vi "Simulated-acquisition-loop.vi"(4 "Timeout":timestamp, 6 "Acquisition notif":refnum<notifier>, 8 "error in (no error)":errorcluster, 9 "Buffers":refnum<class "CV-Buffers.lvclass">, 10 "Config. params. ref. in":refnum<data-value>, 11 "Acquis. params. ref. in":refnum<data-value>) -> (0 "error out":errorcluster, 2 "Config. params. ref.":refnum<data-value>, 3 "Acquis. params. ref.":refnum<data-value>)   [LabVIEW 2013, in "CameraVision.lvlib" / "CV-Acquisition.lvclass"]
uses:
  CV-Acquisition.lvclass
  Configuration/CV-Configuration.lvclass
  Buffers/CV-Buffers.lvclass
  <vilib>/Platform/TimedLoop/XDataNode/timing_clust.ctl
  <vilib>/Platform/TimedLoop/XDataNode/nitl_modes.ctl
  <vilib>/Platform/TimedLoop/XDataNode/wakeup.ctl
  <vilib>/Platform/TimedLoop/XDataNode/XDataNode.xnode
  <vilib>/Platform/TimedLoop/XDataNode/XDNodeRunTimeDep.lvlib
  CV-Main.lvclass
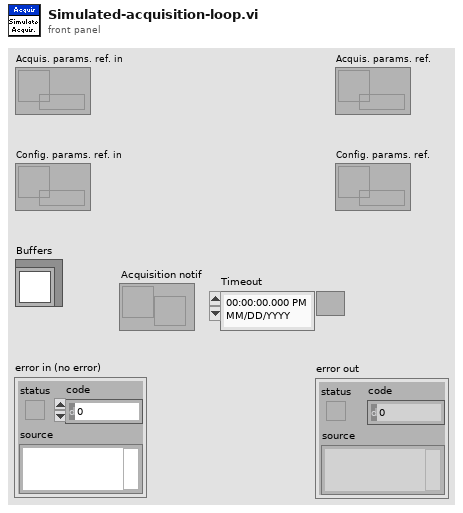
[diagram p1: front panel]
types:
  T1 = typedef "XDNodeRunTimeDep.lvlib/nitl_modes.ctl" = enum32{"No Change", "Process missed periods, maintain original phase", "Discard missed periods, maintain original phase", "Process missed periods, ignore original phase", "Discard missed periods, ignore original phase"}
  T2 = typedef "XDNodeRunTimeDep.lvlib/timing_clust.ctl" = cluster{"Expected End [f-1]":u64, "Actual End [f-1]":u64, "Finished Late? [f-1]":bool, "Expected End [i-1]":u64, "Actual End [i-1]":u64, "Finished Late? [i-1]":bool, "Expected Start [i]":u64, "Actual Start [i]":u64, "Expected Start [f]":u64, "Actual Start [f]":u64, "Source Name":string, "Structure Name":string, "Period":i64, "Deadline":i64, "Offset":i64, "Start":i64, "Priority":i32, "Timeout":i32, "Mode":T1, "Wakeup Reason":T3, "Error":errorcluster, "Source Type":string, "Secondary Source Type":string, "Global End Time":u64, "Global Start Time":u64, "Frame Duration":u64, "Iteration Duration":u64, "Assigned CPU":i32, "I/O Scan Engine Mode":u32}
  T3 = typedef "XDNodeRunTimeDep.lvlib/wakeup.ctl" = enum32{"Normal", "Aborted", "Asynchronous wakeup", "Timing source error", "Timed loop error", "Timeout"}
  T4 = typedef "IMAQ Image.ctl" = refnum<image>
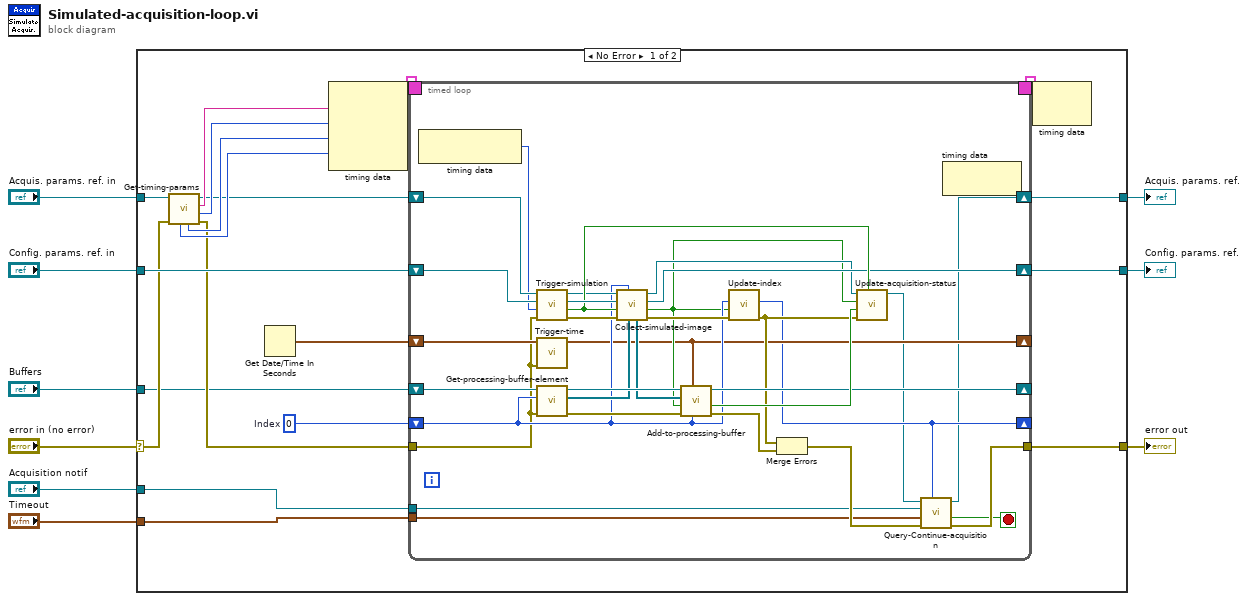
[diagram p0: block diagram]
diagram:
  n1 = case shown="No Error" "error in (no error)" {
    selector: "error in (no error)" -> [w20 w73]
    tunnel: [w17 w73] -> w8
    tunnel: "Acquis. params. ref. in" -> [w24 w72]
    tunnel: [w18 w71] -> w4
    tunnel: [w19 w72] -> w6
    tunnel: "Config. params. ref. in" -> [w21 w71]
    tunnel: "Buffers" -> [w13 _]
    tunnel: "Acquisition notif" -> [w12 _]
    tunnel: "Timeout" -> [w11 _]
    frame No Error {
      w16 = 0  # Index
      n2 = call "Get-timing-params.vi"("error in (no error)"=w20, "Acquis. params. ref. in"=w24) -> ("error out"=w14:errorcluster, "Period"=w26:i64, "Source"=w23:string, "Acquis. params. ref."=w10:refnum<data-value>, "Timeout"=w25:i32, "Mode"=w22:T1)  [unwired: 4 in]
      n3 = Get Date/Time In Seconds() -> (seconds since 1Jan1904=w15:timestamp)
      n4 = node-c288(w23, w26, w25, w22) -> (w28:T2)
      n5 = timed-loop {
        timing: w28 -> [_]
        timing-out: [_] -> w27
        shift-right: [w32] -> w19
        shift-left: w10 -> [w60]
        shift-right: [w48] -> w18
        shift-left: w21 -> [w59]
        shift-right: [w33] -> _
        shift-left: w16 -> [w38]
        shift-right: [w49] -> _
        shift-left: w13 -> [w57]
        tunnel: w14 -> [w35]
        tunnel: [w44] -> w17
        shift-right: [w34] -> _
        shift-left: w15 -> [w36]
        tunnel: w12 -> [w30]
        tunnel: w11 -> [w29]
        stop <- w43 stop-if-true
        n6 = node-c288() -> (w58:T3)  [unwired: 1 in]
        n7 = call "Trigger-simulation.vi"("error in (no error)"=w35, "Wakeup Reason"=w58, "Config. params. ref. in"=w59, "Acquis. params. ref. in"=w60) -> ("error out"=w55:errorcluster, "Tigger ok?"=w51:bool, "Config. params. ref."=w56:refnum<data-value>, "Acquis. params. ref."=w40:refnum<data-value>)  [unwired: 4 in]
        n8 = call "Trigger-time.vi"("error in (no error)"=w35, "Previous time"=w36) -> ("Trigger time"=w34:timestamp)  [unwired: 9 in]
        n9 = call "Get-processing-buffer-element.vi"("error in (no error)"=w35, "Index"=w38, "Buffers in"=w57) -> ("error out"=w53:errorcluster, "Element ref"=w41:T4[], "Buffers out"=w54:refnum<class "CV-Buffers.lvclass">)  [unwired: 6 in]
        n10 = call "Collect-simulated-image.vi"("Images in"=w41, "Index"=w38, "error in (no error)"=w55, "Trigger ok?"=w51, "Config. params. ref. in"=w56, "Acquis. params. ref. in"=w40) -> ("error out"=w52:errorcluster, "Image ok?"=w37:bool, "Config. params. ref."=w48:refnum<data-value>, "Acquis. params. ref."=w39:refnum<data-value>, "Images"=w42:T4[])  [unwired: 1 in]
        n11 = call "Add-to-processing-buffer.vi"("Index"=w38, "Time"=w34, "error in (no error)"=w53, "Image ok?"=w37, "Images"=w42, "Buffers in"=w54) -> ("error out"=w46:errorcluster, "Buffer ok?"=w50:bool, "Buffers out"=w49:refnum<class "CV-Buffers.lvclass">)  [unwired: 3 in]
        n12 = call "Update-index.vi"("error in (no error)"=w52, "Image ok?"=w37, "Index in"=w38) -> ("error out"=w47:errorcluster, "Index"=w33:i32)  [unwired: 7 in]
        n13 = Merge Errors(w47, w46) -> (w45:errorcluster)
        n14 = call "Update-acquisition-status.vi"("Tigger ok?"=w51, "error in (no error)"=w47, "Queue ok?"=w50, "Image ok?"=w37, "Acquis. params. ref. in"=w39) -> ("Acquis. params. ref."=w31:refnum<data-value>)  [unwired: 5 in, 1 out]
        n15 = call "Query-Continue-acquisition.vi"("Index"=w33, "error in"=w45, "Timeout"=w29, "Acquisition notif"=w30, "Acquis. params. ref. in"=w31) -> ("error IO"=w44:errorcluster, "Continue?"=w43:bool, "Acquis. params. ref."=w32:refnum<data-value>)  [unwired: 4 in]
        n16 = node-c288() -> ()  [unwired: 1 in, 1 out]
      }
      n17 = node-c288(w27) -> ()  [unwired: 1 out]
    }
    frame Error {
    }
  }
  "error out" <- w8
  "Acquis. params. ref." <- w6
  "Config. params. ref." <- w4
